vi "Tick Count ms.vi"(8 "error in":errorcluster) -> (0 "error out":errorcluster, 1 "millisecond timer value":u32)   [LabVIEW 2024]
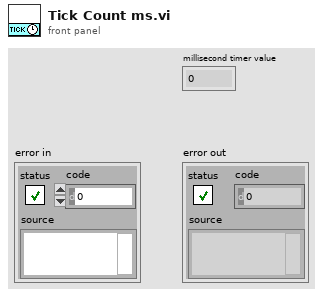
[diagram p1: front panel]
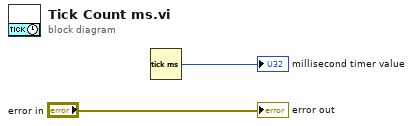
[diagram p0: block diagram]
diagram:
  n1 = Tick Count (ms)() -> (millisecond timer value=→"millisecond timer value":u32)
  "error out" <- "error in"
